vi "BuildServer Launcher.vi"() -> ()   [LabVIEW 2017]
uses:
  Actors/BuildServer/BuildServer/BuildServer.lvclass
  Volumes/Data/Users/benji667/Git/BuildFarm/WebSocket Server/Actors/Actor wHelper/Actor wLauncher/Actor wLauncher.lvclass
  WebSocket Server/Actors/Actor wHelper/Actor wLauncher/Actor wLauncher.lvclass
panel:
  out "Status":string
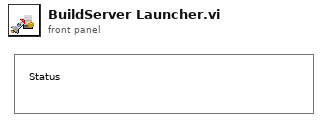
[diagram p1: front panel]
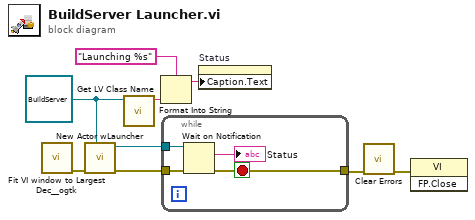
[diagram p0: block diagram]
diagram:
  w8 = refnum<class "BuildServer.lvclass"> refnum ("BuildServer.lvlib:BuildServer.lvclass")
  n1 = call <userlib>:"Fit VI window to Largest Dec__ogtk.vi"() -> ("error out"=w1:errorcluster)  [unwired: 6 in, 1 out]
  n2 = call "New Actor wLauncher.vi"("Actor wLauncher in"=w8, "error in (no error)"=w1) -> ("error out"=w2:errorcluster, "Launcher Notifier"=w9:refnum<notifier>)  [unwired: 7 in, 1 out]
  n3 = call <vilib>:"Get LV Class Name.vi"("object"=w8) -> ("class name"=w7:string)  [unwired: 9 in, 1 out]
  n4 = Format Into String(format string="Launching %s", w7) -> (resulting string=w6:string)  [unwired: 2 in, 1 out]
  n5 = while {
    tunnel: w9 -> [w13]
    tunnel: [w11] -> w4
    tunnel: w2 -> [w10]
    stop <- w11 stop-if-true
    n6 = Wait on Notification(notifier=w13, error in (no error)=w10) -> (notification=→"Status":string, error out=w11:errorcluster)  [unwired: 2 in, 2 out]
  }
  n7 = property on="Status" class="Str"("Caption.Text"=w6) -> ()  [unwired: 2 in, 2 out]
  n8 = call <vilib>:"Clear Errors.vi"("error in (no error)"=w4) -> ("error out"=w3:errorcluster)  [unwired: 5 in, 1 out]
  n9 = invoke class="VI" method="FP.Close"(error in=w3) -> ()  [unwired: 2 in, 3 out]
